vi "Calc PI.vi"() -> ()   [LabVIEW 2025]
uses:
  Number.ctl
panel:
  in  "Animate":bool=TRUE
  in  "Digits":i32=2000
  out "Results":string
  out "(ms)":i32
  out "Status":T1(ring)
  out "Progress":i32(slide) scale=0.0..251.0
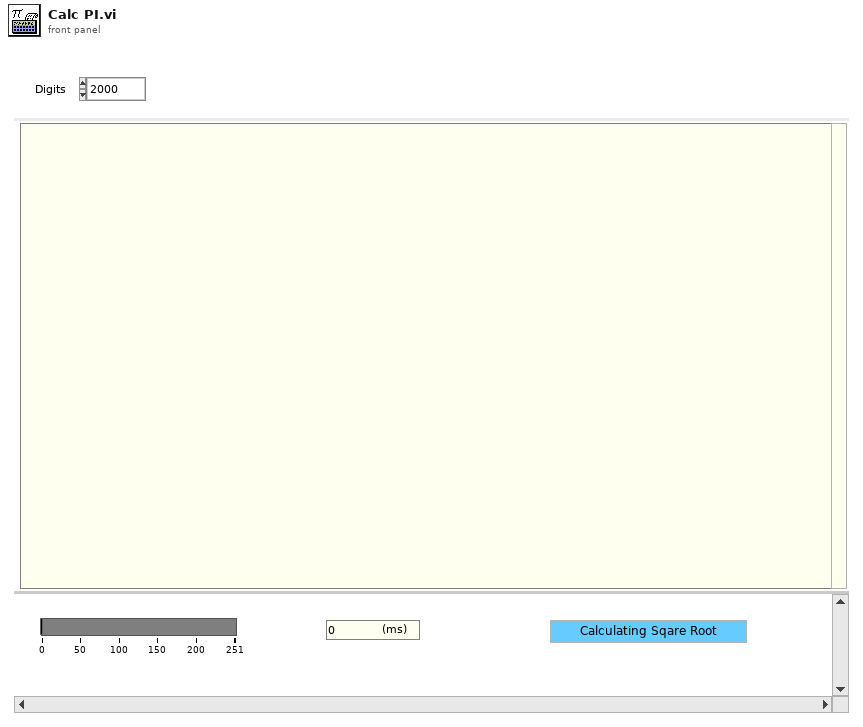
[diagram p1: front panel]
types:
  T1 = enum16{"Calculating Sqare Root", "Iterating Loop", "Finished"}
  T2 = typedef "Number.ctl" = cluster{"Array Num":i8[], "Decimal Index":i32, "stop":bool}
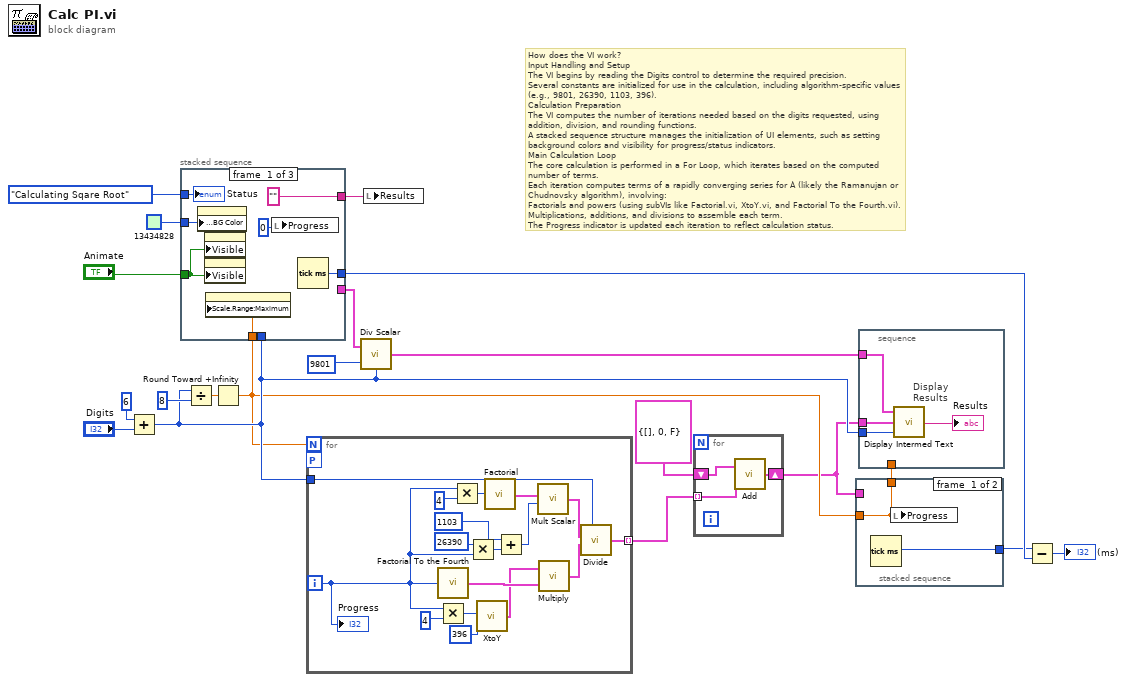
[diagram p0: block diagram]
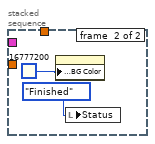
[diagram p2: hidden frame]
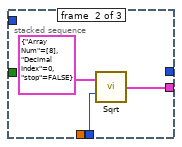
[diagram p3: hidden frame]
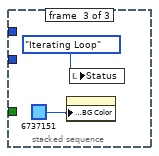
[diagram p4: hidden frame]
diagram:
  # "How does the VI work?\nInput Handling and Setup\nThe VI begins by reading the Digits control to determine the required precision.\nSeveral constants are initialized for use in the calculation, including algorithm-specific values (e.g., 9801, 26390, 1103, 396).\nCalculation Preparation\nThe VI computes the number of iterations needed based on the digits requested, using addition, division, and rounding functions.\nA stacked sequence structure manages the initialization of UI elements, such as setting background colors and visibility for progress/status indicators.\nMain Calculation Loop\nThe core calculation is performed in a For Loop, which iterates based on the computed number of terms.\nEach iteration computes terms of a rapidly converging series for À (likely the Ramanujan or Chudnovsky algorithm), involving:\nFactorials and powers (using subVIs like Factorial.vi, XtoY.vi, and Factorial To the Fourth.vi).\nMultiplications, additions, and divisions to assemble each term.\nThe Progress indicator is updated each iteration to reflect calculation status."
  n1 = Add(x=6 ("digit"), y="Digits") -> (x+y=w6:i32)
  n2 = Divide(x=w6, y=8 ("digit")) -> (x/y=w19:dbl)
  n3 = Round Toward +Infinity(x=w19) -> (ceil(x): smallest int >= x=w5:dbl)
  n4 = stacked-sequence {
    tunnel: w6 -> [_ w30 _]
    tunnel: [_ w29 _] -> w11
    tunnel: T1."Calculating Sqare Root" -> [w27 _ _]
    tunnel: u32 13434828 -> [w26 _ _]
    tunnel: w5 -> [w24 _ _]
    tunnel: [w23 _ _] -> w14
    tunnel: "Animate" -> [w22 _ _]
    tunnel: ["" ("Results") _ _] -> w3
    frame #0 {
      n5 = property on="Status" class="Enum (strict)"("Named Numeric Colors:BG Color"=w26) -> ()  [unwired: 2 in, 2 out]
      n6 = property on="Status" class="Enum (strict)"("Visible"=w22) -> ()  [unwired: 2 in, 2 out]
      n7 = property class="Slide (strict)"("Visible"=w22) -> ()  [unwired: 2 in, 2 out]
      n8 = property class="Slide (strict)"("Scale.Range:Maximum"=w24) -> ()  [unwired: 2 in, 2 out]
      n9 = local write "Progress"(0 ("digit")) -> ()
      n10 = Tick Count (ms)() -> (millisecond timer value=w23:u32)
      "Status" <- w27
    }
    frame #1 {
      n11 = call "Sqrt.vi"("digits"=w30, "A"=T2 {"Array Num"=[8], "Decimal Index"=0, "stop"=FALSE}) -> ("Square Root A"=w29:T2)
    }
    frame #2 {
      n12 = property on="Status" class="Enum (strict)"("Named Numeric Colors:BG Color"=u32 6737151) -> ()  [unwired: 2 in, 2 out]
      n13 = local write "Status"(T1."Iterating Loop") -> ()
    }
  }
  n14 = for {
    N: w5 -> [_]
    tunnel: w6 -> [w49]
    tunnel: [w33] -> w1 mode=indexing
    workers-P: _ -> [_]
    i -> [w48]
    n15 = call "Factorial To the Fourth.vi"("N"=w48) -> ("(N!)^4"=w35:T2)
    n16 = Multiply(x=w48, y=4 ("digit")) -> (x*y=w37:i32)
    n17 = Multiply(x=w48, y=4 ("digit")) -> (x*y=w47:i32)
    n18 = Multiply(x=26390 ("digit"), y=w48) -> (x*y=w43:i32)
    n19 = call "XtoY.vi"("X"=396 ("digit"), "Y"=w37) -> ("Result"=w34:T2)
    n20 = call "Factorial.vi"("N"=w47) -> ("N!"=w40:T2)
    n21 = Add(x=1103 ("digit"), y=w43) -> (x+y=w39:i32)
    n22 = call "Mult Scalar.vi"("A"=w40, "Scalar"=w39) -> ("A x Scalar"=w41:T2)  [unwired: 3 in]
    n23 = call "Multiply.vi"("B"=w35, "A"=w34) -> ("Answer"=w42:T2)
    n24 = call "Divide.vi"("A"=w41, "B"=w42, "digits"=w49) -> ("A/B"=w33:T2)  [unwired: 2 in]
    "Progress" <- w48
  }
  n25 = call "Div Scalar.vi"("Digits"=w6, "Scalar"=9801 ("digit"), "A"=w11) -> ("A / Scalar"=w10:T2)
  n26 = local write "Results"(w3) -> ()
  n27 = for {
    tunnel: w1 -> [w51] mode=indexing
    shift-right: [w52] -> w4
    shift-left: T2 {"Array Num"=[], "Decimal Index"=0, "stop"=FALSE} ("A+B") -> [w50]
    n28 = call "Add.vi"("B"=w51, "A"=w50) -> ("A+B"=w52:T2)
  }
  n29 = stacked-sequence {
    tunnel: [w54 _] -> w13
    tunnel: [w53 _] -> w9
    tunnel: w4 -> [_ _]
    tunnel: w5 -> [w53 _]
    frame #0 {
      n30 = Tick Count (ms)() -> (millisecond timer value=w54:u32)
      n31 = local write "Progress"(w53) -> ()
    }
    frame #1 {
      n32 = property on="Status" class="Enum (strict)"("Named Numeric Colors:BG Color"=u32 16777200) -> ()  [unwired: 2 in, 2 out]
      n33 = local write "Status"(T1."Finished") -> ()
    }
  }
  n34 = stacked-sequence {
    tunnel: w6 -> [w60]
    tunnel: w4 -> [w59]
    tunnel: w10 -> [w58]
    tunnel: w9 -> [_]
    frame #0 {
      # "Display\nResults"
      n35 = call "Display Intermed Text.vi"("A"=w58, "B"=w59, "Digits"=w60) -> ("Results"=→"Results":string)  [unwired: 2 in]
    }
  }
  n36 = Subtract(x=w13, y=w14) -> (x-y=→"(ms)":u32)
